vi "Parse ERD Read Expected Data.vi"(0 "Read ERD List":T1[](array[typedef]) {"ERD Number" format="%.0x"}, 11 "Error In":errorcluster) -> (8 "Expected Data":string, 15 "Error Out":errorcluster)   [LabVIEW 2014, in "GEA2_Toolkit.lvlib"]
uses:
  library/GEA2_Toolkit.lvlib
  type defs/ERD Read Data In.ctl
panel:
  in  "Read ERD List 2":T1[](array[typedef])=[{"ERD Number"=61706, "Data Type"=enum."uint8_t"}, {"ERD Number"=62233, "Data Type"=enum."string"}, {"ERD Number"=61967, "Data Type"=enum."uint16_t"}, {"ERD Number"=61959, "Data Type"=enum."string"}, {"ERD Number"=62219, "Data Type"=enum."uint16_t"}, {"ERD Number"=62221, "Data Type"=enum."uint16_t"}, {"ERD Number"=61953, "Data Type"=enum."uint16_t"}, {"ERD Number"=61954, "Data Type"=enum."uint32_t"}, {"ERD Number"=61708, "Data Type"=enum."uint8_t"}, {"ERD Number"=61963, "Data Type"=enum."uint8_t"}, {"ERD Number"=62237, "Data Type"=enum."uint8_t"}, {"ERD Number"=61961, "Data Type"=enum."uint8_t"}, {"ERD Number"=61968, "Data Type"=enum."string"}, {"ERD Number"=61969, "Data Type"=enum."string"}, {"ERD Number"=61964, "Data Type"=enum."string"}, {"ERD Number"=62227, "Data Type"=enum."uint8_t"}, {"ERD Number"=61971, "Data Type"=enum."string"}, {"ERD Number"=8195, "Data Type"=enum."uint32_t"}, {"ERD Number"=62218, "Data Type"=enum."uint16_t"}, {"ERD Number"=62241, "Data Type"=enum."string"}, {"ERD Number"=61976, "Data Type"=enum."string"}, {"ERD Number"=62243, "Data Type"=enum."string"}, {"ERD Number"=61731, "Data Type"=enum."string"}, {"ERD Number"=61732, "Data Type"=enum."string"}, {"ERD Number"=61698, "Data Type"=enum."string"}, {"ERD Number"=61699, "Data Type"=enum."string"}, {"ERD Number"=61697, "Data Type"=enum."string"}, {"ERD Number"=61704, "Data Type"=enum."string"}, {"ERD Number"=61701, "Data Type"=enum."string"}, {"ERD Number"=61702, "Data Type"=enum."string"}, {"ERD Number"=61705, "Data Type"=enum."string"}, {"ERD Number"=61703, "Data Type"=enum."string"}, {"ERD Number"=61709, "Data Type"=enum."uint16_t"}, {"ERD Number"=61710, "Data Type"=enum."uint16_t"}, {"ERD Number"=61726, "Data Type"=enum."string"}, {"ERD Number"=62213, "Data Type"=enum."uint16_t"}, {"ERD Number"=61952, "Data Type"=enum."uint16_t"}, {"ERD Number"=61957, "Data Type"=enum."uint16_t"}, {"ERD Number"=61958, "Data Type"=enum."uint8_t"}, {"ERD Number"=61973, "Data Type"=enum."uint32_t"}, {"ERD Number"=62242, "Data Type"=enum."string"}, {"ERD Number"=256, "Data Type"=enum."string"}, {"ERD Number"=61441, "Data Type"=enum."string"}, {"ERD Number"=61457, "Data Type"=enum."string"}, {"ERD Number"=61995, "Data Type"=enum."uint16_t"}, {"ERD Number"=61985, "Data Type"=enum."uint16_t"}, {"ERD Number"=61986, "Data Type"=enum."uint16_t"}, {"ERD Number"=65535, "Data Type"=enum."string"}, {"ERD Number"=65535, "Data Type"=enum."string"}, {"ERD Number"=65535, "Data Type"=enum."string"}, {"ERD Number"=61977, "Data Type"=enum."string"}, {"ERD Number"=61990, "Data Type"=enum."string"}, {"ERD Number"=61988, "Data Type"=enum."uint16_t"}, {"ERD Number"=61987, "Data Type"=enum."uint16_t"}, {"ERD Number"=61989, "Data Type"=enum."uint16_t"}, {"ERD Number"=61991, "Data Type"=enum."string"}, {"ERD Number"=62212, "Data Type"=enum."uint16_t"}, {"ERD Number"=62211, "Data Type"=enum."uint16_t"}, {"ERD Number"=62210, "Data Type"=enum."uint16_t"}, {"ERD Number"=62208, "Data Type"=enum."uint16_t"}, {"ERD Number"=62253, "Data Type"=enum."uint16_t"}, {"ERD Number"=62213, "Data Type"=enum."uint16_t"}, {"ERD Number"=62254, "Data Type"=enum."uint16_t"}, {"ERD Number"=62209, "Data Type"=enum."uint16_t"}, {"ERD Number"=61962, "Data Type"=enum."string"}, {"ERD Number"=62229, "Data Type"=enum."string"}, {"ERD Number"=62214, "Data Type"=enum."string"}, {"ERD Number"=62215, "Data Type"=enum."string"}, {"ERD Number"=62230, "Data Type"=enum."string"}, {"ERD Number"=62216, "Data Type"=enum."string"}, {"ERD Number"=62231, "Data Type"=enum."string"}, {"ERD Number"=61760, "Data Type"=enum."uint32_t"}] {"ERD Number" format="%.0x"}
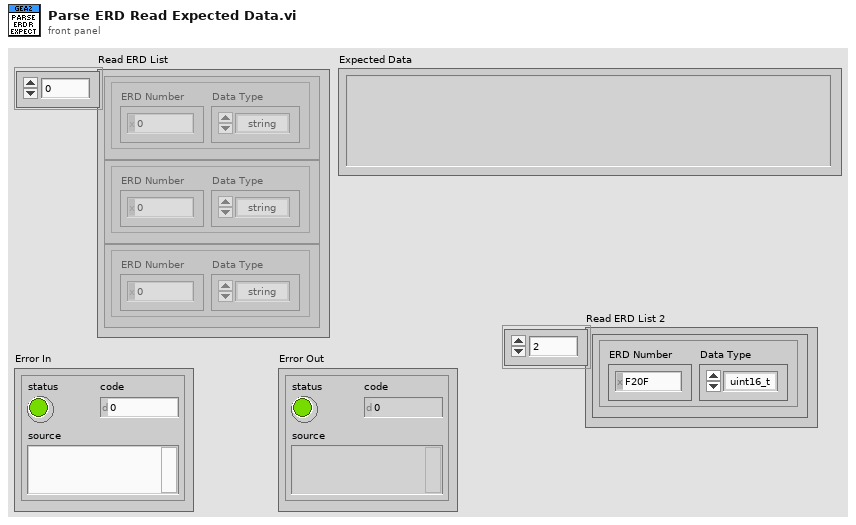
[diagram p1: front panel]
types:
  T1 = typedef "GEA2_Toolkit.lvlib/ERD Read Data In.ctl" = cluster{"ERD Number":u16, "Data Type":enum16{"string", "boolean", "uint8_t", "uint16_t", "uint32_t", "uint64_t"}}
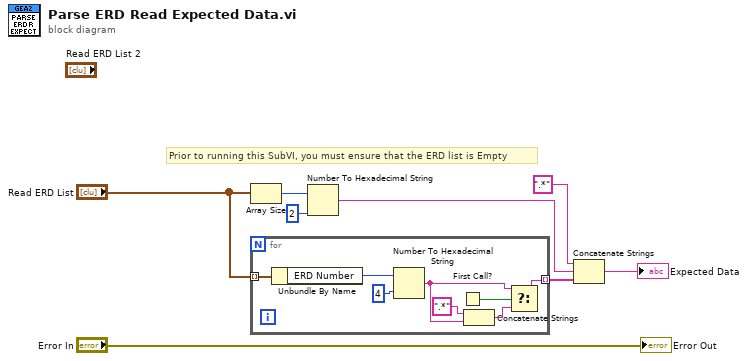
[diagram p0: block diagram]
diagram:
  # "Prior to running this SubVI, you must ensure that the ERD list is Empty"
  n1 = Array Size(array="Read ERD List") -> (size(s)=w5:i32)
  n2 = for {
    tunnel: "Read ERD List" -> [w16] mode=indexing
    tunnel: [w9] -> w6 mode=indexing
    n3 = Unbundle By Name(w16) -> ("ERD Number"=w15:u16)
    n4 = Number To Hexadecimal String(1:i16 4 ("width (-)"), 2:w15) -> (0:w10:string)
    n5 = First Call?() -> (First Call?: T/F=w12:bool)
    n6 = Concatenate Strings(".*" ("string"), w10) -> (w11:string)
    n7 = Select(t=w10, s=w12, f=w11) -> (s? t:f=w9:string)
  }
  n8 = Number To Hexadecimal String(1:i16 2 ("width (-)"), 2:w5) -> (0:w3:string)
  n9 = Concatenate Strings(".*" ("string"), w3, w6) -> (→"Expected Data":string)
  "Error Out" <- "Error In"
